vi "Check-Mapping-settings.vi"(8 "error in":errorcluster, 9 "Temp. params. ref.":refnum<data-value>, 10 "Analysis params. ref.":refnum<data-value>, 11 "Mapping params. ref.":refnum<data-value>) -> (0 "error IO":errorcluster, 3 "Passed?":bool)   [LabVIEW 2013, in "CameraVision.lvlib" / "CV-Mapping.lvclass"]
uses:
  CV-Mapping.lvclass
  Temperature/CV-Temperature.lvclass
  Analysis/CV-Analysis.lvclass
  Analysis/CV-Analysis.lvclass/CV-Analysis.ctl
  CV-Mapping.lvclass/CV-Mapping.ctl
  Temperature/CV-Temperature.lvclass/CV-Temperature.ctl
  Read Enable mapping.vi
  Analysis/Read Image characteristics.vi
  Analysis/Read Melt-pool characteristics.vi
  Temperature/Read Temperature value.vi
  Write Available.vi
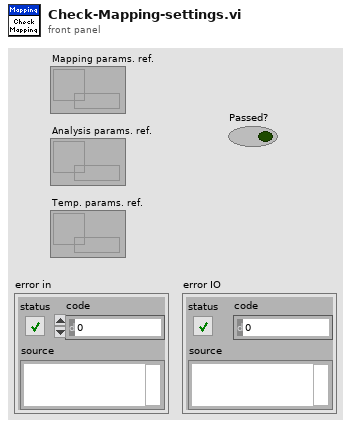
[diagram p1: front panel]
types:
  T1 = typedef "CameraVision.lvlib/CV-Mapping.lvclass/Mapping-characteristic.ctl" = enum16{"Average intensity [0-255]", "Peak intensity [0-255]", "Melt-pool size [mm²]", "Melt-pool aspect ratio []", "Melt-pool fragments []", "Average temperature [°C]", "Max. temperature [°C]", "Min. temperature [°C]", "Std. dev. temperature [°C]"}
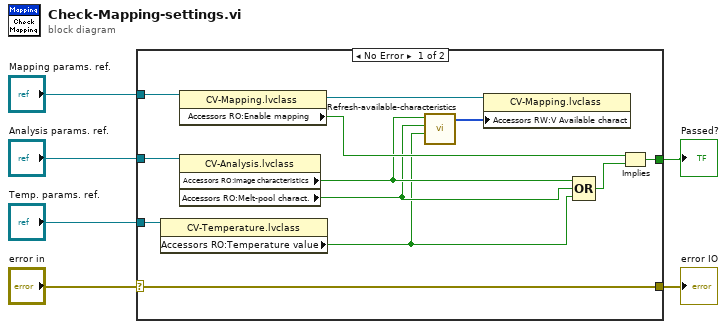
[diagram p0: block diagram]
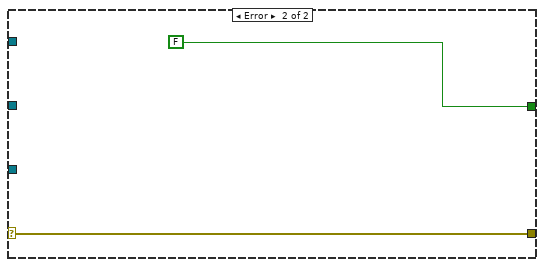
[diagram p2: hidden frame]
diagram:
  n1 = case shown="No Error" "error in" {
    selector: "error in" -> [w11 w19]
    tunnel: "Temp. params. ref." -> [w13 _]
    tunnel: [w11 w19] -> w5
    tunnel: [w18 FALSE] -> w6
    tunnel: "Mapping params. ref." -> [w16 _]
    tunnel: "Analysis params. ref." -> [w14 _]
    frame No Error {
      n2 = property class="CV-Temperature.lvclass"(reference=w13) -> ("Accessors RO:Temperature value"=w7:bool)  [unwired: 1 in, 2 out]
      n3 = property class="CV-Mapping.lvclass"(reference=w16) -> (reference out=w12:refnum<data-value>, "Accessors RO:Enable mapping"=w15:bool)  [unwired: 1 in, 1 out]
      n4 = property class="CV-Analysis.lvclass"(reference=w14) -> ("Accessors RO:Image characteristics"=w9:bool, "Accessors RO:Melt-pool charact."=w8:bool)  [unwired: 1 in, 2 out]
      n5 = call "Refresh-available-characteristics.vi"("Temperature value"=w7, "Melt-pool charact"=w8, "Image characteristics"=w9) -> ("Available"=w10:T1[])  [unwired: 7 in, 1 out]
      n6 = property class="CV-Mapping.lvclass"(reference=w12, "Accessors RW:V Available charact"=w10) -> ()  [unwired: 1 in, 2 out]
      n7 = Compound Arithmetic op=OR(w9, w8, w7) -> (w17:bool)
      n8 = Implies(1:w17, 2:w15) -> (0:w18:bool)
    }
    frame Error {
    }
  }
  "Passed?" <- w6
  "error IO" <- w5
